vi "Lockin.DAQ.Read AI and Write AO.vi"(8 "error in (no error)":errorcluster, 10 "AO []":waveform(dbl)[](array[waveform]), 11 "Lockin.DAQ in":refnum<class "Lockin.DAQ.lvclass">) -> (0 "error out":errorcluster, 1 "AO []":waveform(dbl)[](array[waveform]), 2 "AI []":waveform(dbl)[](array[waveform]), 3 "Lockin.DAQ out":refnum<class "Lockin.DAQ.lvclass">)   [LabVIEW 2016, in "Lockin.DAQ.lvclass"]
uses:
  Lockin.DAQ.lvclass
panel:
  out "AO":u32
  out "AI":u32
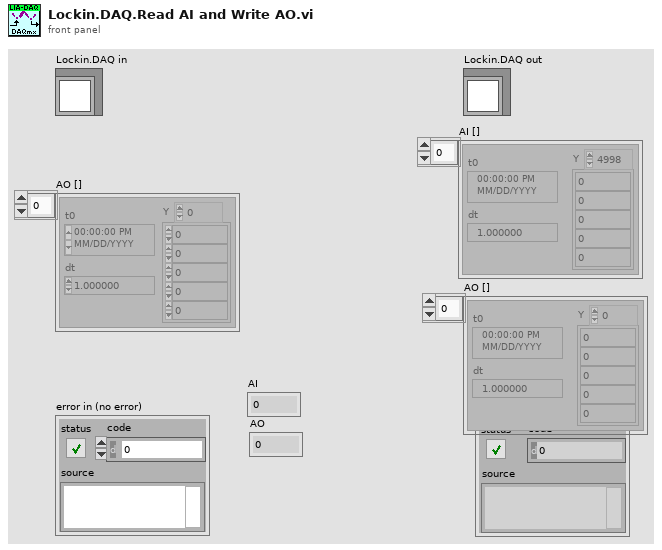
[diagram p1: front panel]
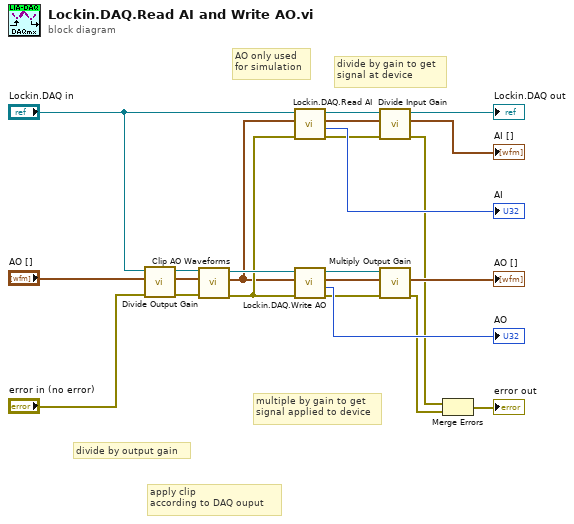
[diagram p0: block diagram]
diagram:
  # "divide by gain to get\nsignal at device"
  # "multiple by gain to get\nsignal applied to device"
  # "apply clip\naccording to DAQ ouput"
  # "divide by output gain"
  # "AO only used\nfor simulation"
  n1 = call "Divide Output Gain.vi"("error in (no error)"="error in (no error)", "WFM in"="AO []", "Lockin.DAQ"="Lockin.DAQ in") -> ("error out"=w17:errorcluster, "WFM out"=w19:waveform(dbl)[], "Lockin.DAQ out"=w18:refnum<class "Lockin.DAQ.lvclass">)  [unwired: 6 in]
  n2 = call "Clip AO Waveforms.vi"("error in (no error)"=w17, "AO []"=w19, "Lockin.DAQ in"=w18) -> ("error out"=w15:errorcluster, "Clipped AO []"=w1:waveform(dbl)[], "Lockin.DAQ out"=w16:refnum<class "Lockin.DAQ.lvclass">)  [unwired: 6 in]
  n3 = call "Lockin.DAQ.Read AI.vi"("error in (no error)"=w15, "AO []"=w1, "Lockin.DAQ in"="Lockin.DAQ in") -> ("error out"=w9:errorcluster, "AI time (ms)"=→"AI":u32, "AI []"=w11:waveform(dbl)[], "Lockin.DAQ out"=w10:refnum<class "Lockin.DAQ.lvclass">)  [unwired: 5 in]
  n4 = call "Lockin.DAQ.Write AO.vi"("error in (no error)"=w15, "AO []"=w1, "Lockin.DAQ in"=w16) -> ("error out"=w8:errorcluster, "AO time (ms)"=→"AO":u32, "AO out []"=w6:waveform(dbl)[], "Lockin.DAQ out"=w13:refnum<class "Lockin.DAQ.lvclass">)  [unwired: 5 in]
  n5 = call "Divide Input Gain.vi"("error in (no error)"=w9, "WFM in"=w11, "Lockin.DAQ"=w10) -> ("error out"=w4:errorcluster, "WFM out"=→"AI []":waveform(dbl)[], "Lockin.DAQ out"=→"Lockin.DAQ out":refnum<class "Lockin.DAQ.lvclass">)  [unwired: 6 in]
  n6 = call "Multiply Output Gain.vi"("error in (no error)"=w8, "WFM in"=w6, "Lockin.DAQ"=w13) -> ("error out"=w3:errorcluster, "WFM out"=→"AO []":waveform(dbl)[])  [unwired: 6 in, 1 out]
  n7 = Merge Errors(w4, w3) -> (→"error out":errorcluster)
